vi "Write username.vi"(8 "error in (no error)":errorcluster, 10 "username":string, 11 "URI in":refnum<class "URI.lvclass">) -> (0 "error out":errorcluster, 3 "URI out":refnum<class "URI.lvclass">)   [LabVIEW 2013, in "openURI.lvlib" / "URI.lvclass"]
uses:
  URI.lvclass
  URI.lvclass/URI.ctl
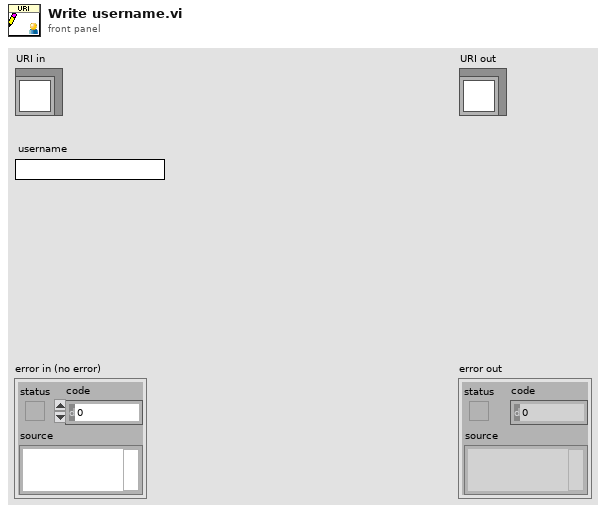
[diagram p1: front panel]
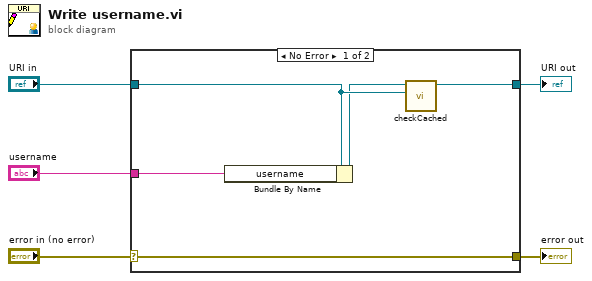
[diagram p0: block diagram]
diagram:
  n1 = case shown="No Error" "error in (no error)" {
    selector: "error in (no error)" -> [w10 w11]
    tunnel: [w10 w11] -> w4
    tunnel: [w6 w12] -> w2
    tunnel: "URI in" -> [w8 w12]
    tunnel: "username" -> [w9 _]
    frame No Error {
      n2 = Bundle By Name(cluster=w8, "username"=w9) -> (w7:refnum<class "URI.lvclass">)
      n3 = call "checkCached.vi"("Old"=w8, "New URI"=w7) -> ("URI"=w6:refnum<class "URI.lvclass">)  [unwired: 9 in]
    }
    frame Error {
    }
  }
  "error out" <- w4
  "URI out" <- w2
